vi "Set NVM Settings.vi"(0 "reference in":refnum<class "Stand.lvclass">, 5 "data":T1, 11 "error in (no error)":errorcluster) -> (4 "reference out":refnum<class "Stand.lvclass">, 15 "error out":errorcluster)   [LabVIEW 2019, in "Stand.lvclass"]
uses:
  Stand.lvclass
  modbus engine custom/MB_ENGINE_class/MB_ENGINE.lvclass
  NeedleValve_class/NeedleValve.lvclass
  TypeDef/Needle Valve Settings.ctl
  modbus engine custom/MB_ENGINE_class/Settings.ctl
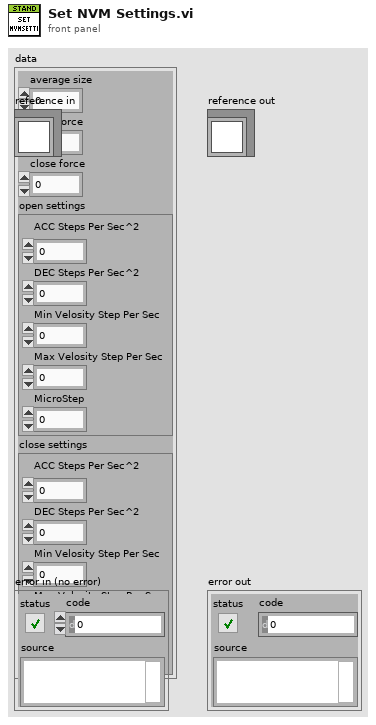
[diagram p1: front panel]
types:
  T1 = typedef "Needle Valve Settings.ctl" = cluster{"average size":i32, "open force":u16, "close force":u16, "open settings":T2, "close settings":T2}
  T2 = typedef "MB_ENGINE.lvclass/Settings.ctl" = cluster{"ACC Steps Per Sec^2":u16, "DEC Steps Per Sec^2":u16, "Min Velosity Step Per Sec":u16, "Max Velosity Step Per Sec":u16, "MicroStep":u16}
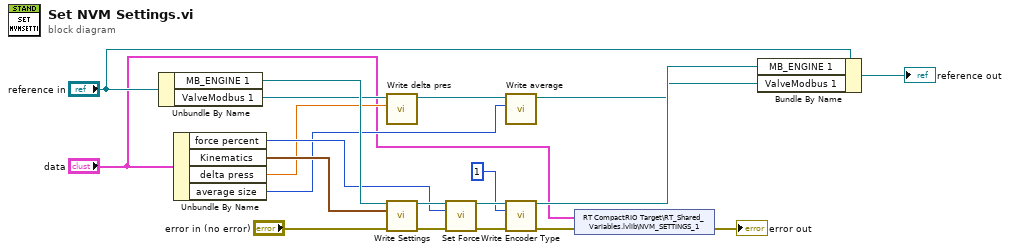
[diagram p0: block diagram]
diagram:
  n1 = Unbundle By Name("reference in") -> ("MB_ENGINE 1"=w15:refnum<class "MB_ENGINE.lvclass">, "ValveModbus 1"=w7:refnum<class "NeedleValve.lvclass">)
  n2 = Unbundle By Name("data") -> ("force percent"=w13:u16, "Kinematics"=w16:T2, "delta press"=w9:dbl, "average size"=w8:i32)
  n3 = call "Write delta pres.vi"("delta pres"=w9, "ValveModbus in"=w7) -> ("ValveModbus out"=w6:refnum<class "NeedleValve.lvclass">)  [unwired: 9 in]
  n4 = call-dynamic "Write Settings.vi"("class data in"=w15, "cluster"=w16, "error in (no error)"="error in (no error)") -> ("class data out"=w20:refnum<class "MB_ENGINE.lvclass">, "error out"=w14:errorcluster)  [unwired: 11 in]
  n5 = call-dynamic "Set Force.vi"("class data in"=w20, "percent"=w13, "error in (no error)"=w14) -> ("class data out"=w19:refnum<class "MB_ENGINE.lvclass">, "error out"=w18:errorcluster)  [unwired: 11 in]
  n6 = call "Write average.vi"("average"=w8, "ValveModbus in"=w6) -> ("ValveModbus out"=w5:refnum<class "NeedleValve.lvclass">)  [unwired: 9 in]
  n7 = call-dynamic "Write Encoder Type.vi"("class data in"=w19, "U16"=u16 1, "error in (no error)"=w18) -> ("class data out"=w11:refnum<class "MB_ENGINE.lvclass">, "error out"=w2:errorcluster)  [unwired: 11 in]
  n8 = shared-variable "RT CompactRIO Target\\RT_Shared_Variables.lvlib\\NVM_SETTINGS_1"("data", error in=w2) -> (error out=→"error out":errorcluster)
  n9 = Bundle By Name(cluster="reference in", "MB_ENGINE 1"=w11, "ValveModbus 1"=w5) -> (→"reference out":refnum<class "Stand.lvclass">)
